vi "Init Messaging.vi"(8 "error in (no error)":errorcluster, 11 "LV Chat Server in":refnum<class "LV Chat Server.lvclass">) -> (0 "error out":errorcluster, 3 "LV Chat Server out":refnum<class "LV Chat Server.lvclass">)   [LabVIEW 2020, in "LV Chat Server.lvclass"]
uses:
  LV Chat Server.lvclass
  <vilib>/IlluminatedG/lv-stream-tcp/TCP Server/TCP Server.lvclass
  C:/Program Files (x86)/National Instruments/LabVIEW 2020/vi.lib/IlluminatedG/lv-stream/Endpoint/Endpoint.lvclass
  Data Types/Message ID.ctl
  LV Chat Server.lvclass/LV Chat Server.ctl
  4c5b7ff5-26a5-498c-a58b-ae976ed6ec19.vi
  9f5becab-4deb-49ae-acb6-8af2dfbfa484.vi
  User Info Message Callback.vi
  Chat Message Callback.vi
  Connection Callback.vi
  <vilib>/IlluminatedG/lv-stream/Endpoint/Endpoint.lvclass
  Stream-Simple-Msg/Manager/Manager.lvclass
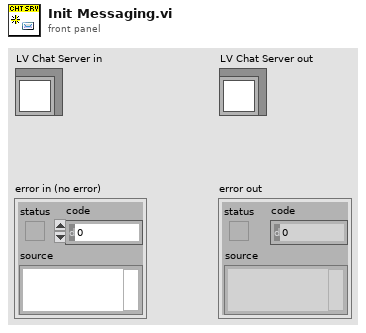
[diagram p1: front panel]
types:
  T1 = typedef "Message ID.ctl" = enum16{"UserInfo", "UserList", "Message", "Disconnect"}
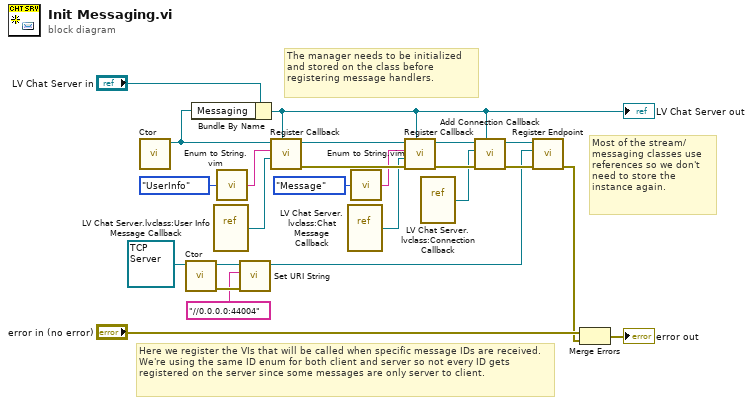
[diagram p0: block diagram]
diagram:
  # "Most of the stream/messaging classes use references so we don't need to store the instance again."
  # "Here we register the VIs that will be called when specific message IDs are received. We're using the same ID enum for both client and server so not every ID gets registered on the server since some messages are only server to client."
  # "The manager needs to be initialized and stored on the class before registering message handlers."
  n1 = call "Ctor.vi"() -> ("Manager out"=w2:refnum<class "Manager.lvclass">)  [unwired: 10 in, 1 out]
  n2 = call-dynamic "Ctor.vi"("TCP Server in"=refnum<class "TCP Server.lvclass"> refnum) -> ("error out"=w17:errorcluster, "TCP Server out"=w18:refnum<class "TCP Server.lvclass">)  [unwired: 9 in]
  n3 = Bundle By Name(cluster="LV Chat Server in", "Messaging"=w2) -> (w7:refnum<class "LV Chat Server.lvclass">)
  "LV Chat Server out" <- w7
  n4 = vi-ref "LV Chat Server.lvclass:User Info Message Callback.vi"() -> (w13:refnum<vi>)
  n5 = call "Enum to String.vim"("Enum"=Message_ID."UserInfo" ("Message ID")) -> ("Enum String"=w14:string)
  n6 = call <vilib>:"Set URI String.vi"("error in (no error)"=w17, "URI String"="//0.0.0.0:44004", "Endpoint in"=w18) -> ("Endpoint out"=w5:refnum<class "TCP Server.lvclass">)  [unwired: 7 in, 1 out]
  n7 = call "Register Callback.vi"("Owner"=w7, "Callback"=w13, "Message ID"=w14, "Manager in"=w2) -> ("error out"=w22:errorcluster, "Manager out"=w9:refnum<class "Manager.lvclass">)  [unwired: 6 in]
  n8 = vi-ref "LV Chat Server.lvclass:Chat Message Callback.vi"() -> (w12:refnum<vi>)
  n9 = call "Enum to String.vim"("Enum"=Message_ID."Message" ("Message ID")) -> ("Enum String"=w11:string)
  n10 = call "Register Callback.vi"("Owner"=w7, "error in (no error)"=w22, "Callback"=w12, "Message ID"=w11, "Manager in"=w9) -> ("error out"=w23:errorcluster, "Manager out"=w3:refnum<class "Manager.lvclass">)  [unwired: 5 in]
  n11 = vi-ref "LV Chat Server.lvclass:Connection Callback.vi"() -> (w6:refnum<vi>)
  n12 = call "Add Connection Callback.vi"("Owner"=w7, "error in (no error)"=w23, "Callback"=w6, "Manager in"=w3) -> ("error out"=w24:errorcluster, "Manager out"=w1:refnum<class "Manager.lvclass">)  [unwired: 6 in]
  n13 = call "Register Endpoint.vi"("error in (no error)"=w24, "Stream:Endpoint"=w5, "Manager in"=w1) -> ("error out"=w4:errorcluster)  [unwired: 7 in, 1 out]
  n14 = Merge Errors("error in (no error)", w4) -> (→"error out":errorcluster)
